vi "Video_WriteFrameBuffer.vi"(11 "Frame Buffers":T1) -> (0 "error out":errorcluster)   [LabVIEW 2020]
uses:
  Controls/Raycaster_DrawState.ctl
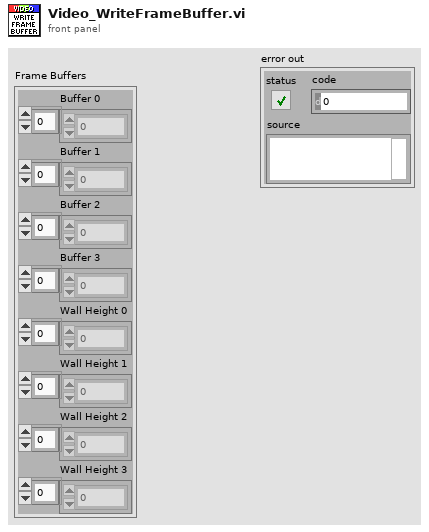
[diagram p1: front panel]
types:
  T1 = typedef "Raycaster_DrawState.ctl" = cluster{"Buffer 0":u8[], "Buffer 1":u8[], "Buffer 2":u8[], "Buffer 3":u8[], "Wall Height 0":i16[], "Wall Height 1":i16[], "Wall Height 2":i16[], "Wall Height 3":i16[]}
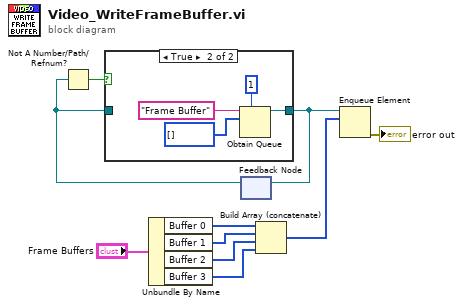
[diagram p0: block diagram]
diagram:
  n1 = Unbundle By Name("Frame Buffers") -> ("Buffer 0"=w6:u8[], "Buffer 1"=w5:u8[], "Buffer 2"=w4:u8[], "Buffer 3"=w3:u8[])
  n2 = feedback #1() -> (w8:refnum<queue>)  [unwired: 1 in]
  n3 = Not A Number/Path/Refnum?(number/path/refnum=w8) -> (NaN/Path/Refnum?=w10:bool)
  n4 = case shown="True" w10 {
    tunnel: [w11 w12] -> w9
    tunnel: w8 -> [w11 _]
    frame False {
    }
    frame True {
      n5 = Obtain Queue(max queue size (-1, unlimited)=1, name (unnamed)="Frame Buffer", element data type=u8[] [] ("Frame Buffer")) -> (queue out=w12:refnum<queue>)  [unwired: 2 in, 2 out]
    }
  }
  n6 = feedback-in #1(w9) -> ()
  n7 = Build Array (concatenate)(w6, w5, w4, w3) -> (w2:u8[])
  n8 = Enqueue Element(queue=w9, element=w2) -> (error out=→"error out":errorcluster)  [unwired: 2 in, 2 out]
